vi "E1A_Checksum.vi"(11 "Data":u8[](array[numeric])) -> (3 "Checksum":bool)   [LabVIEW 2022 SP3]
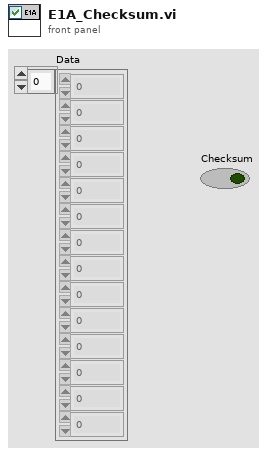
[diagram p1: front panel]
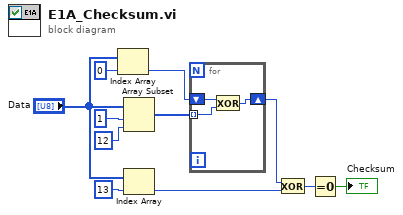
[diagram p0: block diagram]
diagram:
  n1 = Index Array(array="Data", index=0) -> (element=w9:u8)
  n2 = Array Subset(array="Data", index=1 ("length"), length=12 ("index")) -> (w10:u8[])
  n3 = Index Array(array="Data", index=13) -> (element=w3:u8)
  n4 = for {
    shift-right: [w12] -> w4
    shift-left: w9 -> [w14]
    tunnel: w10 -> [w13] mode=indexing
    n5 = Exclusive Or(1:w13, 2:w14) -> (0:w12:u8)
  }
  n6 = Exclusive Or(1:w3, 2:w4) -> (0:w2:u8)
  n7 = Equal To 0?(x=w2) -> (x = 0?=→"Checksum":bool)
